vi "STM_Client_OO_2.vi"() -> ()   [LabVIEW 2016, in "RemoteControl.STM.lvclass"]
uses:
  RemoteControl.STM.lvclass
  <vilib>/NI/STM/SubVIs/MetaDataElement.ctl
  RemoteControl.STM.lvclass/RemoteControl.STM.ctl
  <userlib>/_OpenG.lib/error/error.llb/Filter Error Codes (Array)__ogtk.vi
  <vilib>/NI/STM/NI STM.lvlib
panel:
  out "startup time (ms)":u32
  out "messsages/s":dbl
  in  "remote port":u16=6341
  in  "address":string
  out "Data reponse":variant
  out "time (ms)":u32
  out "Numeric":i32
  in  "Data":string
  in  "stop":bool
  out "Command reponse":string
  in  "Command":string
  out "meta data\n(available commands)":T1[](array[typedef])
  out "error out":errorcluster
  # "CLIENT (API)"
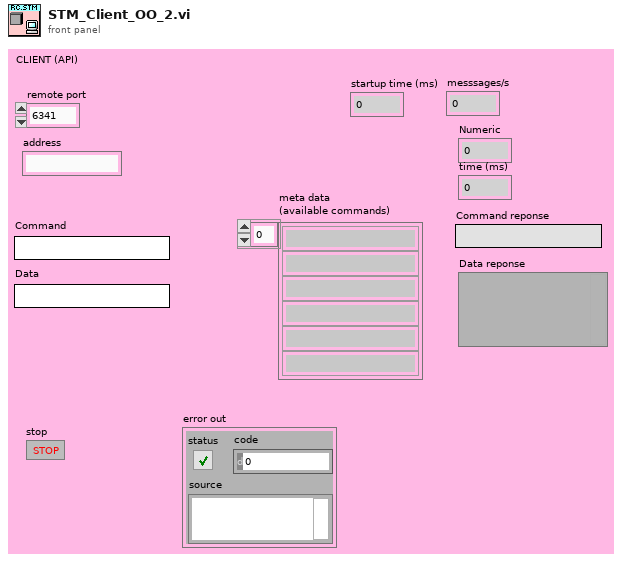
[diagram p1: front panel]
types:
  T1 = typedef "NI STM.lvlib/MetaDataElement.ctl" = string
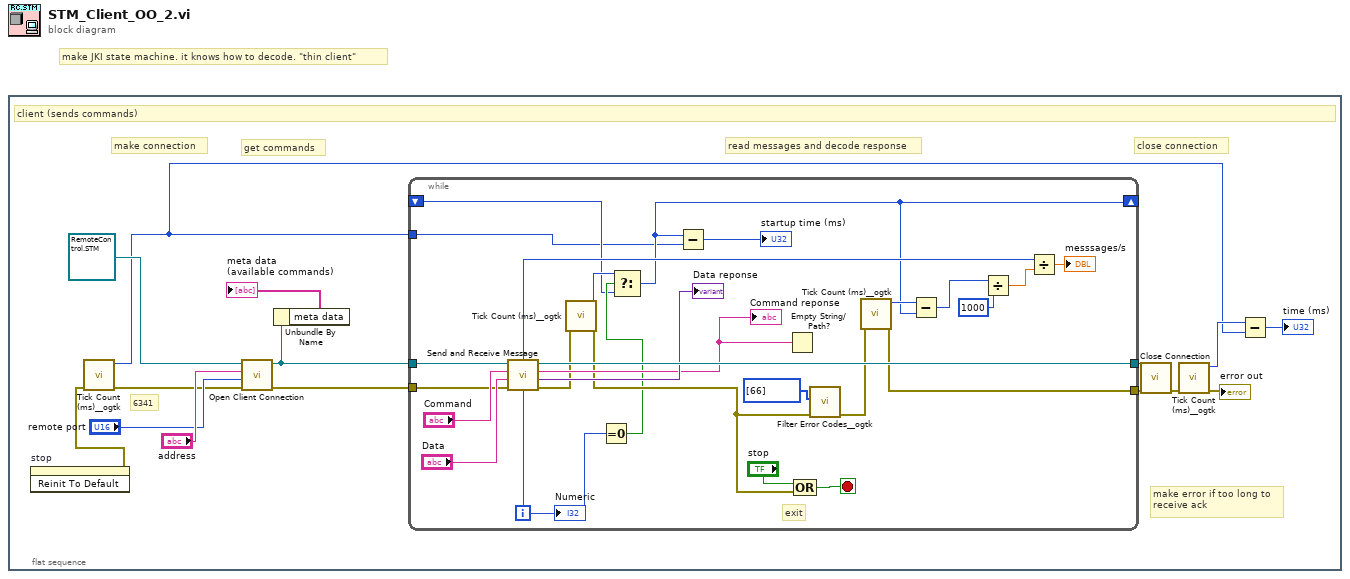
[diagram p0: block diagram]
diagram:
  # "make JKI state machine. it knows how to decode. \"thin client\""
  n1 = flat-sequence {
    frame #0 {
      # "close connection"
      # "read messages and decode response"
      # "get commands"
      # "make connection"
      # "6341"
      # "make error if too long to\nreceive ack"
      # "client (sends commands)"
      n2 = invoke on="stop" class="Bool (strict)" method="Reinit To Default"() -> (error out=w12:errorcluster)  [unwired: 3 in, 2 out]
      n3 = call <userlib>:"Tick Count (ms)__ogtk.vi"("error in (no error)"=w12) -> ("error out"=w4:errorcluster, "millisecond timer value"=w1:u32)  [unwired: 9 in]
      n4 = call-dynamic "Open Client Connection.vi"("error in (no error)"=w4, "Port"="remote port", "address"="address", "RemoteControl.STM in"=refnum<class "RemoteControl.STM.lvclass"> refnum) -> ("error out"=w2:errorcluster, "RemoteControl.STM out"=w7:refnum<class "RemoteControl.STM.lvclass">)  [unwired: 6 in]
      n5 = Unbundle By Name(w7) -> ("meta data"=→"meta data\n(available commands)":T1[])
      n6 = while {
        tunnel: [w31] -> w15
        tunnel: [w37] -> w14
        tunnel: w2 -> [w33]
        tunnel: w7 -> [w38]
        tunnel: w1 -> [w16]
        shift-right: [w17] -> _
        shift-left: _ -> [w18]
        i -> [w19]
        stop <- w41 stop-if-true
        # "exit"
        n7 = call-dynamic "Send and Receive Message.vi"("error in (no error)"=w33, "Data"="Data", "Command"="Command", "RemoteControl in"=w38) -> ("error out"=w24:errorcluster, "Data out"=→"Data reponse":variant, "Command out"=w26:string, "RemoteControl out"=w37:refnum<class "RemoteControl.STM.lvclass">)  [unwired: 4 in]
        "Command reponse" <- w26
        n8 = call <userlib>:"Tick Count (ms)__ogtk.vi"("error in (no error)"=w24) -> ("error out"=w23:errorcluster, "millisecond timer value"=w21:u32)  [unwired: 9 in]
        n9 = Equal To 0?(x=w19) -> (x = 0?=w20:bool)
        n10 = Select(t=w21, s=w20, f=w18) -> (s? t:f=w17:u32)
        n11 = Subtract(x=w17, y=w16) -> (x-y=→"startup time (ms)":u32)
        n12 = Empty String/Path?(string/path=w26) -> ()  [unwired: 1 out]
        n13 = Compound Arithmetic op=OR("stop", w23) -> (w41:bool)
        n14 = call-poly <userlib>:"Filter Error Codes__ogtk.vi"("Error In"=w23, "Error Codes to Filter"=i32[] [66]) -> ("Error Out"=w32:errorcluster)  [unwired: 7 in, 2 out]
        n15 = call <userlib>:"Tick Count (ms)__ogtk.vi"("error in (no error)"=w32) -> ("error out"=w31:errorcluster, "millisecond timer value"=w25:u32)  [unwired: 9 in]
        n16 = Subtract(x=w25, y=w17) -> (x-y=w28:u32)
        n17 = Divide(x=w28, y=u32 1000) -> (x/y=w30:dbl)
        n18 = Divide(x=w19, y=w30) -> (x/y=→"messsages/s":dbl)
        "Numeric" <- w19
      }
      n19 = call-dynamic "Close Connection.vi"("error in (no error)"=w15, "RemoteControl.STM in"=w14) -> ("error out"=w13:errorcluster)  [unwired: 8 in, 1 out]
      n20 = call <userlib>:"Tick Count (ms)__ogtk.vi"("error in (no error)"=w13) -> ("error out"=→"error out":errorcluster, "millisecond timer value"=w10:u32)  [unwired: 9 in]
      n21 = Subtract(x=w10, y=w1) -> (x-y=→"time (ms)":u32)
    }
  }
